vi "Remove Selected Items From Lists.vi"(10 "SelectedItems":i32[](array[numeric]), 11 "ListBox Tests In":T1) -> (1 "Deleted CSV(s)":path[](array[path]), 3 "ListBox Tests In Out":T1)   [LabVIEW 2011]
uses:
  Controls/ListBox Test Record.ctl
  <userlib>/_OpenG.lib/array/array.llb/Delete Elements from 1D Array (String)__ogtk.vi
  <userlib>/_OpenG.lib/array/array.llb/Delete Elements from 1D Array (Path)__ogtk.vi
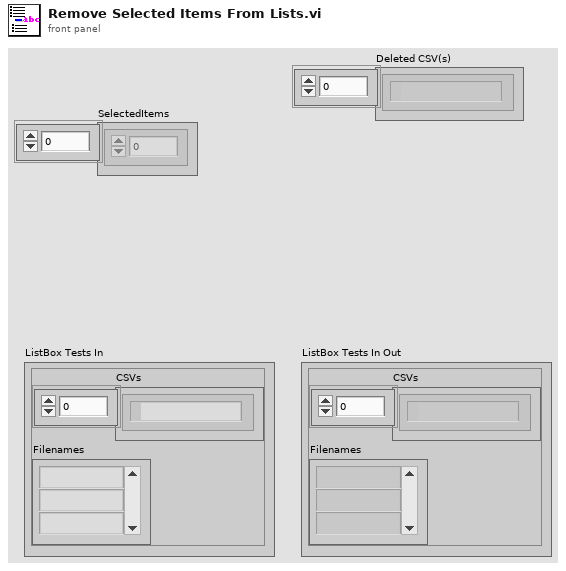
[diagram p1: front panel]
types:
  T1 = typedef "ListBox Test Record.ctl" = cluster{"CSVs":path[], "Filenames":string[]}
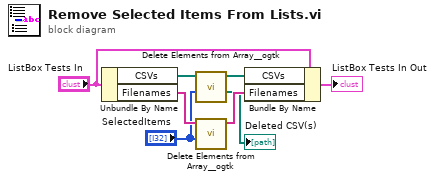
[diagram p0: block diagram]
diagram:
  n1 = Unbundle By Name("ListBox Tests In") -> ("CSVs"=w4:path[], "Filenames"=w6:string[])
  n2 = call-poly <userlib>:"Delete Elements from Array__ogtk.vi"("indices"="SelectedItems", "array"=w4) -> ("deleted elements"=→"Deleted CSV(s)":path[], "array w/ subset deleted"=w3:path[])  [unwired: 8 in]
  n3 = call-poly <userlib>:"Delete Elements from Array__ogtk.vi"("indices"="SelectedItems", "array"=w6) -> ("array w/ subset deleted"=w5:string[])  [unwired: 8 in, 1 out]
  n4 = Bundle By Name(cluster="ListBox Tests In", "CSVs"=w3, "Filenames"=w5) -> (→"ListBox Tests In Out":T1)
